vi "Mass Compile.vi"(8 "error in (no error)":errorcluster, 11 "Path Filter":string) -> (0 "error out":errorcluster)   [LabVIEW 2013]
doc: "Performs a mass compile of all files located in immediate sub directories of the <vilib>\\LapDog\\Messaging directory where the file path includes the text defined by Path Filter.\n\ne.g.\n<vilib>\\LapDog\\Messaging\\FilterMatch is mass compiled.\n<vilib>\\LapDog\\Messaging\\OtherDirectory\\FilterMatch is not mass compiled.\n\nCreates a log file located in ProgramData\\LapDog\\logs\\mclog.txt"
uses:
  <vilib>/Utility/sysdir.llb/System Directory Type.ctl
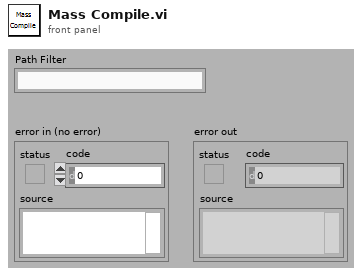
[diagram p1: front panel]
types:
  T1 = typedef "System Directory Type.ctl" = i32
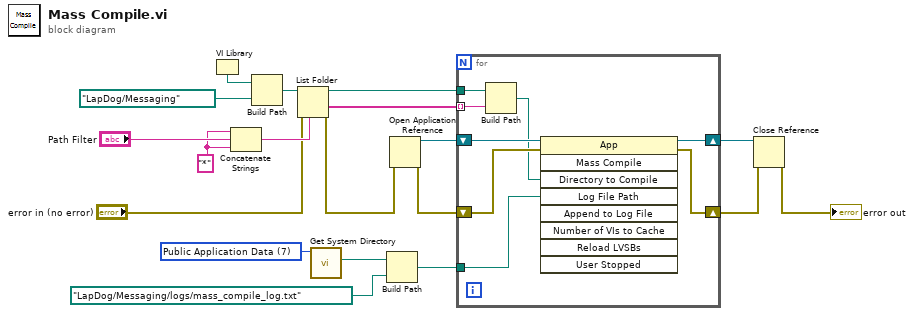
[diagram p0: block diagram]
diagram:
  w7 = T1 7 items=["User Home", "User Desktop", "User Documents", "User Application Data", "User Preferences", "User Temporary", "Public Documents", "Public Application Data", "Public Preferences", "System Core Libraries", "System Installed Libraries", "Application Files", "Boot Volume Root"] ("system directory type")
  w17 = "*"
  n1 = VI Library() -> (path=w3:path)
  n2 = Concatenate Strings(w17, "Path Filter", w17) -> (w18:string)
  n3 = Build Path(base path=w3, name or relative path=path "LapDog/Messaging") -> (appended path=w1:path)
  n4 = List Folder(path=w1, pattern=w18, error in="error in (no error)") -> (path out=w8:path, folder names=w9:string[], error out=w14:errorcluster)  [unwired: 1 in, 1 out]
  n5 = call <vilib>:"Get System Directory.vi"("system directory type"=w7) -> ("system directory"=w6:path)  [unwired: 10 in]
  n6 = Build Path(base path=w6, name or relative path=path "LapDog/Messaging/logs/mass_compile_log.txt" ("Log File Path")) -> (appended path=w4:path)
  n7 = Open Application Reference(8:w14) -> (0:w13:errorcluster, 3:w15:refnum<vi>)  [unwired: 3 in]
  n8 = for {
    tunnel: w9 -> [w23] mode=indexing
    shift-right: [w26] -> w11
    shift-left: w13 -> [w27]
    shift-right: [w24] -> w12
    shift-left: w15 -> [w25]
    tunnel: w8 -> [w22]
    tunnel: w4 -> [w20]
    n9 = Build Path(base path=w22, name or relative path=w23) -> (appended path=w21:path)
    n10 = invoke class="App" method="Mass Compile"(reference=w25, error in=w27, "Directory to Compile"=w21, "Log File Path"=w20) -> (reference out=w24:refnum<vi>, error out=w26:errorcluster)  [unwired: 5 in, 7 out]
  }
  n11 = Close Reference(reference=w12, error in (no error)=w11) -> (error out=→"error out":errorcluster)
